vi "Handle Error.vi"(8 "error in (no error)":errorcluster, 11 "Camera in":refnum<class "Camera.lvclass">) -> (0 "error out":errorcluster, 2 "stop actor?":bool=TRUE, 3 "Camera out":refnum<class "Camera.lvclass">)   [LabVIEW 2021, in "Camera.lvlib" / "Camera.lvclass"]
doc: "(<B>Filename</B>: Actor Framework.lvlib:Actor.lvclass:Handle Error.vi)\n\nDefines how the actor handles an error that occurred while processing a message. By default, this method does nothing except stop the actor."
uses:
  Camera.lvclass
  <vilib>/ActorFramework/Actor/Actor.lvclass
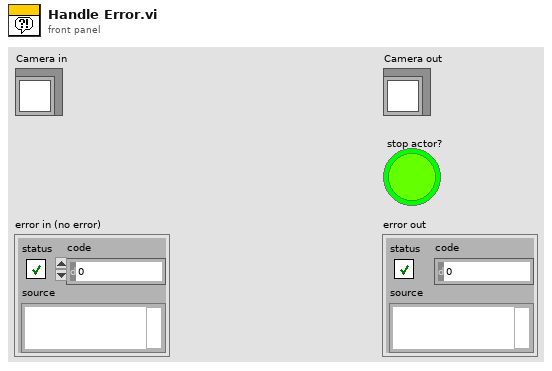
[diagram p1: front panel]
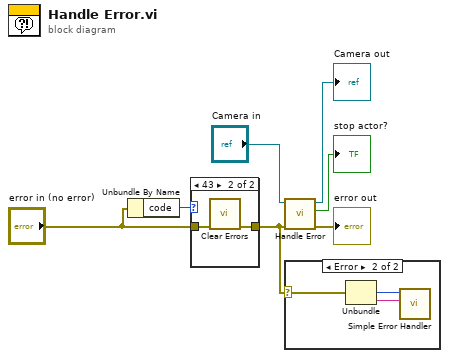
[diagram p0: block diagram]
diagram:
  n1 = Unbundle By Name("error in (no error)") -> ("code"=w3:i32)
  n2 = case shown="43" w3 {
    tunnel: "error in (no error)" -> [w8 w10]
    tunnel: [w8 w9] -> w1
    frame Default {
    }
    frame 43 {
      n3 = call <vilib>:"Clear Errors.vi"("error in (no error)"=w10) -> ("error out"=w9:errorcluster)  [unwired: 5 in, 1 out]
    }
  }
  n4 = call-parent "Handle Error.vi"("error in (no error)"=w1, "Actor in"="Camera in") -> ("error out"=→"error out":errorcluster, "stop actor?"=→"stop actor?":bool, "Actor out"=→"Camera out":refnum<class "Camera.lvclass">)  [unwired: 7 in]
  n5 = case shown="Error" w1 {
    selector: w1 -> [_ w13]
    frame No Error {
    }
    frame Error {
      n6 = Unbundle(w13) -> ("code"=w12:i32, "source"=w11:string)  [unwired: 1 out]
      n7 = call <vilib>:"Simple Error Handler.vi"("error code (no error:0)"=w12, "error source (\" \")"=w11) -> ()  [unwired: 3 in, 5 out]
    }
  }
